vi "Calc - RPMPercent.vi"(11 "00-03-9402(RPM)":dbl[](array[numeric])) -> (2 "N2%":dbl, 3 "N1%":dbl)   [LabVIEW 2018, in "Controller (Host).lvlib"]
uses:
  Controller (Host).lvlib
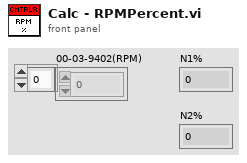
[diagram p1: front panel]
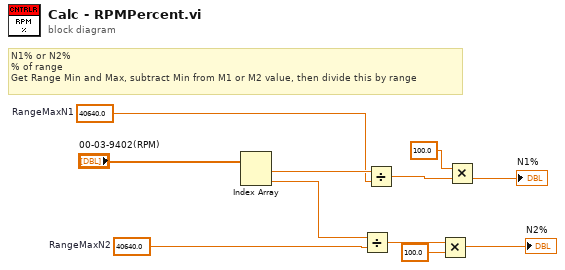
[diagram p0: block diagram]
diagram:
  w7 = 40640.0  # RangeMaxN2
  w9 = 40640.0  # RangeMaxN1
  # "N1% or N2%\n% of range\nGet Range Min and Max, subtract Min from M1 or M2 value, then divide this by range"
  n1 = Index Array(array="00-03-9402(RPM)") -> (element #1=w10:dbl, element #2=w6:dbl)  [unwired: 2 in]
  n2 = Divide(x=w6, y=w7) -> (x/y=w5:dbl)
  n3 = Divide(x=w10, y=w9) -> (x/y=w8:dbl)
  n4 = Multiply(x=w5, y=100.0) -> (x*y=→"N2%":dbl)
  n5 = Multiply(x=100.0, y=w8) -> (x*y=→"N1%":dbl)
